vi "TouchPanel.formatNumber.vi"(0 "number in":ext format="%#_25g", 2 "show all digits (F)":bool, 11 "significant digits (6)":i16=6, 13 "Integer (F)":bool) -> (4 "number out":ext format="%#_25g", 8 "string out":string, 15 "DB string out":string)   [LabVIEW 2016]
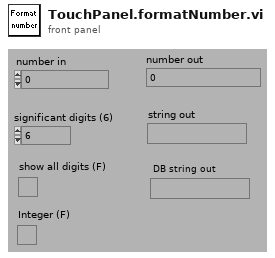
[diagram p1: front panel]
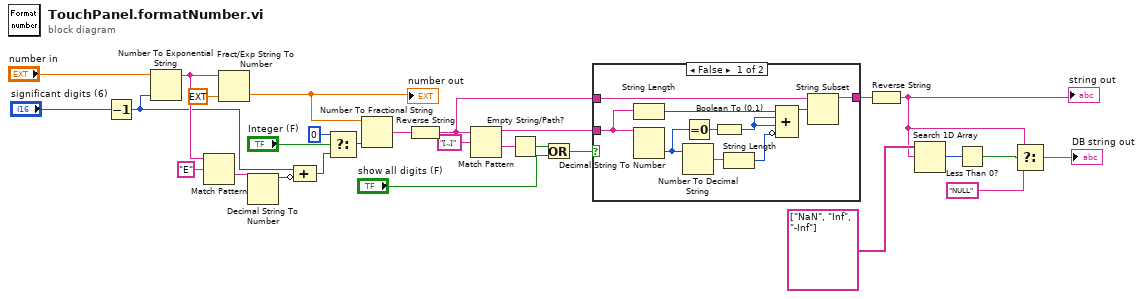
[diagram p0: block diagram]
diagram:
  n1 = Decrement(x="significant digits (6)") -> (x-1=w22:i16)
  n2 = Number To Exponential String(number="number in", precision (6)=w22) -> (E-format string=w26:string)  [unwired: 1 in, 1 out]
  n3 = Match Pattern(string=w26, regular expression="E") -> (after substring=w24:string)  [unwired: 4 out]
  n4 = Fract/Exp String To Number(string=w26, default (0 dbl)=ext 0.0 ("number in")) -> (number=w27:ext)  [unwired: 1 in, 2 out]
  "number out" <- w27
  n5 = Decimal String To Number(string=w24) -> (number=w21:i32)  [unwired: 3 out]
  n6 = Compound Arithmetic op=ADD(w22, invert w21) -> (w3:i32)
  n7 = Select(t=0, s="Integer (F)", f=w3) -> (s? t:f=w2:i32)
  n8 = Number To Fractional String(number=w27, precision (6)=w2) -> (F-format string=w19:string)  [unwired: 1 in, 1 out]
  n9 = Reverse String(1:w19) -> (0:w18:string)
  n10 = Match Pattern(string=w18, regular expression="[.,]") -> (before substring=w16:string, after substring=w15:string)  [unwired: 3 out]
  n11 = Empty String/Path?(string/path=w15) -> (empty?=w14:bool)
  n12 = Or(x=w14, y="show all digits (F)") -> (x .or. y?=w13:bool)
  n13 = case shown="False" w13 {
    tunnel: w18 -> [w37 w39]
    tunnel: [w36 w39] -> w17
    tunnel: w16 -> [w35 _]
    frame False {
      n14 = String Length(string=w35) -> (length=w32:i32)
      n15 = Decimal String To Number(string=w35) -> (number=w34:i32)  [unwired: 3 out]
      n16 = Number To Decimal String(number=w34) -> (decimal integer string=w38:string)  [unwired: 1 out]
      n17 = Equal To 0?(x=w34) -> (x = 0?=w30:bool)
      n18 = Boolean To (0,1)(Boolean=w30) -> (0, 1=w29:i16)
      n19 = String Length(string=w38) -> (length=w31:i32)
      n20 = Compound Arithmetic op=ADD(w32, w29, w29, invert w31) -> (w33:i32)
      n21 = String Subset(string=w37, offset (0)=w33) -> (substring=w36:string)  [unwired: 1 out]
    }
    frame True {
    }
  }
  n22 = Reverse String(1:w17) -> (0:w6:string)
  "string out" <- w6
  n23 = Search 1D Array(1D array=string[] ["NaN", "Inf", "-Inf"], element=w6) -> (index of element=w11:i32)  [unwired: 1 out]
  n24 = Less Than 0?(x=w11) -> (x < 0?=w10:bool)
  n25 = Select(t=w6, s=w10, f="NULL") -> (s? t:f=→"DB string out":string)
